vi "Validate_Destination.vi"(8 "error in (no error)":errorcluster, 10 "Destination":refnum<class "AB_Destination.lvclass">, 11 "AB_Source in":refnum<class "AB_Source.lvclass">) -> (0 "error out":errorcluster, 2 "Valid":bool, 3 "AB_Source out":refnum<class "AB_Source.lvclass">)   [LabVIEW 2020, in "AB_Source.lvclass"]
uses:
  <vilib>/AppBuilder/AB_Classes/Source/AB_Source.lvclass
  <vilib>/AppBuilder/AB_Classes/Destination/AB_Destination.lvclass
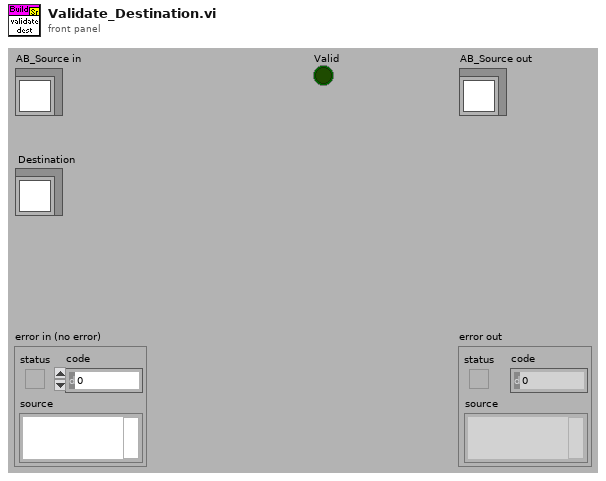
[diagram p1: front panel]
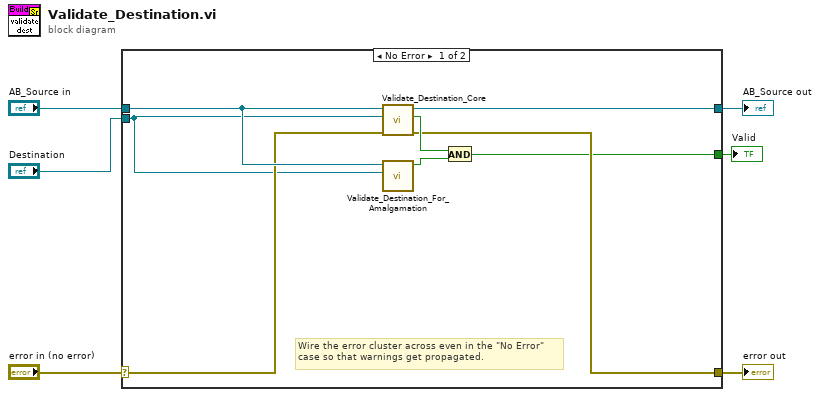
[diagram p0: block diagram]
diagram:
  n1 = case shown="No Error" "error in (no error)" {
    selector: "error in (no error)" -> [w10 w16]
    tunnel: [w9 w16] -> w5
    tunnel: [w13 w15] -> w3
    tunnel: "AB_Source in" -> [w14 w15]
    tunnel: [w8 _] -> w2
    tunnel: "Destination" -> [w7 _]
    frame No Error {
      # "Wire the error cluster across even in the \"No Error\"\ncase so that warnings get propagated."
      n2 = call-dynamic "Validate_Destination_Core.vi"("error in (no error)"=w10, "Destination"=w7, "AB_Source in"=w14) -> ("error out"=w9:errorcluster, "valid"=w12:bool, "AB_Source out"=w13:refnum<class "AB_Source.lvclass">)  [unwired: 6 in]
      n3 = call <vilib>:"Validate_Destination_For_Amalgamation.vi"("Destination"=w7, "AB_Source.lvclass"=w14) -> ("Valid?"=w11:bool)  [unwired: 9 in]
      n4 = And(x=w12, y=w11) -> (x .and. y?=w8:bool)
    }
    frame Error {
    }
  }
  "error out" <- w5
  "AB_Source out" <- w3
  "Valid" <- w2
